vi "Get Result Obj by Type.vi"(8 "error in (no error)":errorcluster, 10 "Parameter Type":refnum<class "Analyze Results Base.lvclass">, 11 "Analyze BaseClass in":refnum<class "Analyze BaseClass.lvclass">) -> (0 "error out":errorcluster, 1 "found?":bool, 2 "Parameter":refnum<class "Analyze Results Base.lvclass">, 3 "Analyze BaseClass out":refnum<class "Analyze BaseClass.lvclass">)   [LabVIEW 2020, in "Analyze.lvlib" / "Analyze BaseClass.lvlib" / "Analyze BaseClass.lvclass"]
uses:
  Analyze BaseClass.lvclass
  Results and Overlays/Results Base/Analyze Results Base.lvclass
  Analyze BaseClass.lvclass/Analyze BaseClass.ctl
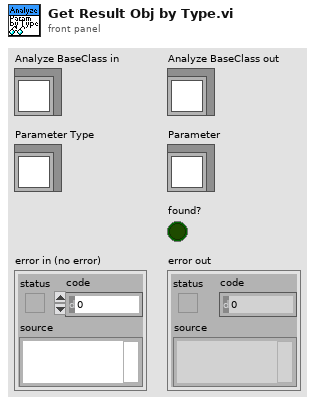
[diagram p1: front panel]
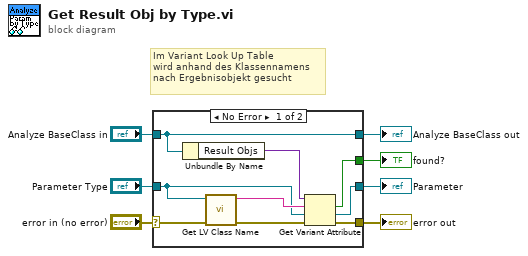
[diagram p0: block diagram]
diagram:
  # "Im Variant Look Up Table\nwird anhand des Klassennamens\nnach Ergebnisobjekt gesucht"
  n1 = case shown="No Error" "error in (no error)" {
    selector: "error in (no error)" -> [w10 w19]
    tunnel: [w8 w19] -> w6
    tunnel: [w16 w18] -> w4
    tunnel: "Analyze BaseClass in" -> [w16 w18]
    tunnel: "Parameter Type" -> [w13 w17]
    tunnel: [w12 w17] -> w2
    tunnel: [w11 _] -> w1
    frame No Error {
      n2 = Unbundle By Name(w16) -> ("Result Objs"=w15:variant)
      n3 = call <vilib>:"Get LV Class Name.vi"("error in (no error)"=w10, "object"=w13) -> ("error out"=w9:errorcluster, "class name"=w14:string)  [unwired: 8 in]
      n4 = Get Variant Attribute(Variant=w15, name=w14, default value (empty Variant)=w13, error in=w9) -> (found=w11:bool, value=w12:refnum<class "Analyze Results Base.lvclass">, error out=w8:errorcluster)  [unwired: 1 out]
    }
    frame Error {
    }
  }
  "error out" <- w6
  "Analyze BaseClass out" <- w4
  "Parameter" <- w2
  "found?" <- w1
